vi "_DServerGetAttributeInfo.vi"(3 "error in":errorcluster, 4 "attribute name":string, 5 "device name":string) -> (0 "error out":errorcluster, 1 "attribute info":T1)   [LabVIEW 2014, in "tango.lvlib"]
uses:
  tango.lvlib
  tango_binding.so
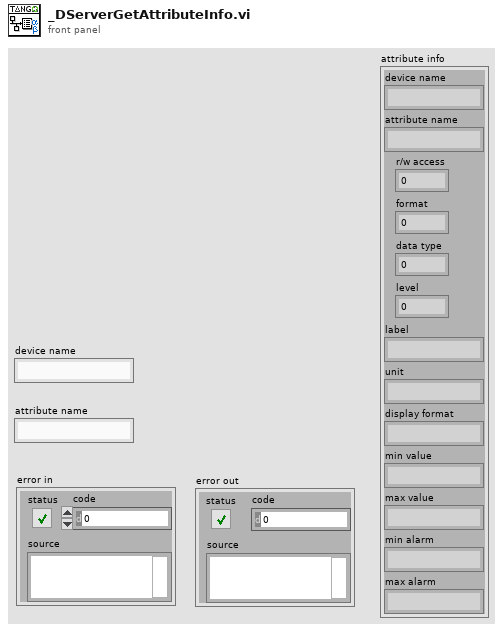
[diagram p1: front panel]
types:
  T1 = cluster{"device name":string, "attribute name":string, "r/w access":i16, "format":i16, "data type":i16, "level":i16, "label":string, "unit":string, "display format":string, "min value":string, "max value":string, "min alarm":string, "max alarm":string}
  T2 = typedef "tango.lvlib/_AttributeInfo_t.ctl" = cluster{"device name":string, "attribute name":string, "r/w access":T3, "format":T4, "data type":T5, "level":T6, "label":string, "unit":string, "display format":string, "min value":string, "max value":string, "min alarm":string, "max alarm":string}
  T3 = typedef "tango.lvlib/_AttributeAccess_t.ctl" = enum16{"READ", "READ_WITH_WRITE", "WRITE", "READ_WRITE", "UNKNOWN_ACCESS_TYPE"}
  T4 = typedef "tango.lvlib/_AttributeFormat_t.ctl" = enum16{"SCALAR", "SPECTRUM", "IMAGE", "UNKNOWN_FORMAT"}
  T5 = typedef "tango.lvlib/_TangoDataType_t.ctl" = enum16{"VOID", "BOOLEAN", "SHORT", "LONG", "FLOAT", "DOUBLE", "USHORT", "ULONG", "STRING", "CHAR_ARRAY", "SHORT_ARRAY", "LONG_ARRAY", "FLOAT_ARRAY", "DOUBLE_ARRAY", "USHORT_ARRAY", "ULONG_ARRAY", "STRING_ARRAY", "LONG_STRING_ARRAY", "DOUBLE_STRING_ARRAY", "STATE", "CONST_STRING", "BOOLEAN_ARRAY", "UCHAR", "LONG64", "ULONG64", "LONG64_ARRAY", "ULONG64_ARRAY", "INT (not supported)", "ENCODED (not supported)", "ENUM", "PIPE_BLOB (not supported)", "STATE_ARRAY", "UNKNOW_DATA_TYPE"}
  T6 = typedef "tango.lvlib/_AttributeLevel_t.ctl" = enum16{"OPERATOR", "EXPERT", "UNKNOWN_LEVEL"}
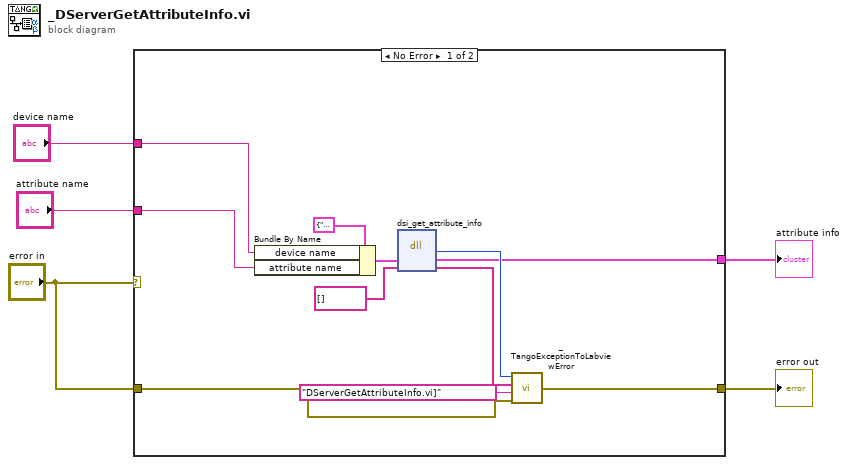
[diagram p0: block diagram]
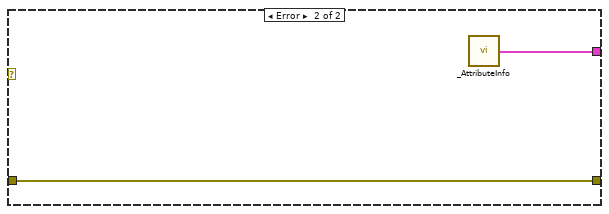
[diagram p2: hidden frame]
diagram:
  n1 = case shown="No Error" "error in" {
    tunnel: [w15 w18] -> w4
    tunnel: "error in" -> [w14 w18]
    tunnel: [w7 w17] -> w3
    tunnel: "device name" -> [w9 _]
    tunnel: "attribute name" -> [w8 _]
    frame No Error {
      n2 = Bundle By Name(cluster=T1 {"device name"="", "attribute name"="", "r/w access"=0, "format"=0, "data type"=0, "level"=0, "label"="", "unit"="", "display format"="", "min value"="", "max value"="", "min alarm"="", "max alarm"=""}, "device name"=w9, "attribute name"=w8) -> (w6:T1)
      n3 = dll-call lib="tango_binding.*" fn="dsi_get_attribute_info"("attrs_info_inout"=w6, "error_stack"=string[] [] ("error stack")) -> ("return type"=w11:i32, "attrs_info_inout"=w7:T1, "error_stack"=w12:string[])  [unwired: 3 in, 2 out]
      n4 = call "_TangoExceptionToLabviewError.vi"("error in"=w14, "location"="DServerGetAttributeInfo.vi]", "error stack"=w12, "error code"=w11) -> ("error out"=w15:errorcluster)
    }
    frame Error {
      n5 = call "_AttributeInfo.vi"() -> ("attribute info"=w17:T2)  [unwired: 15 in]
    }
  }
  "error out" <- w4
  "attribute info" <- w3
